vi "readEthernetLimitsFromXml.vi"(6 "type":string, 8 "error in (no error)":errorcluster, 9 "device.lvclass":refnum<class "device.lvclass">, 10 "xml in":refnum<class "NativeXML.lvclass">, 11 "deviceDataBase in":refnum<class "deviceDataBase.lvclass">) -> (0 "error out":errorcluster, 1 "device.lvclass out":refnum<class "device.lvclass">, 2 "xml out":refnum<class "NativeXML.lvclass">, 3 "deviceDataBase out":refnum<class "deviceDataBase.lvclass">)   [LabVIEW 2009, in "Tools.lvlib" / "DatabaseHelpers.lvlib" / "deviceDataBase.lvclass"]
uses:
  deviceDataBase.lvclass
  Database Objects/device/device.lvclass
  NativeXML/NativeXML.lvclass
  Database Objects/device/EthernetSupply/ethernetSupply.lvclass
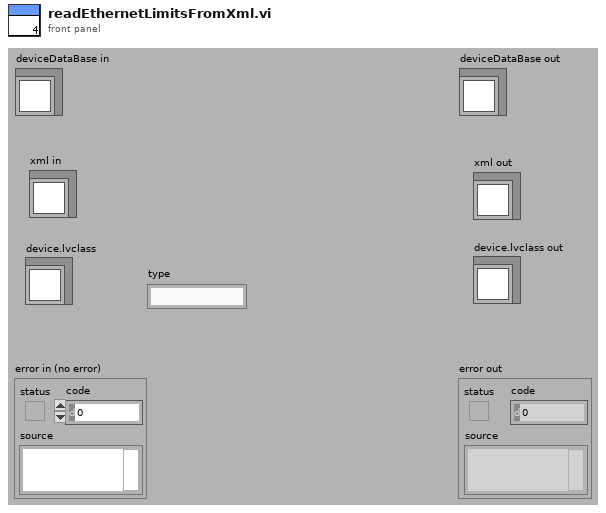
[diagram p1: front panel]
types:
  T1 = cluster{"Range":cluster{"units":string, "min":dbl, "max":dbl}, "triggering_inUse":cluster{"start_trigger":string, "clock":string}, "Limits":cluster{"VoltageLimit":dbl, "CurrentLimit":dbl}}[]
  T2 = cluster{"Range":cluster{"units":string, "min":dbl, "max":dbl}, "triggering_inUse":cluster{"start_trigger":string, "clock":string}, "Limits":cluster{"VoltageLimit":dbl, "CurrentLimit":dbl}}
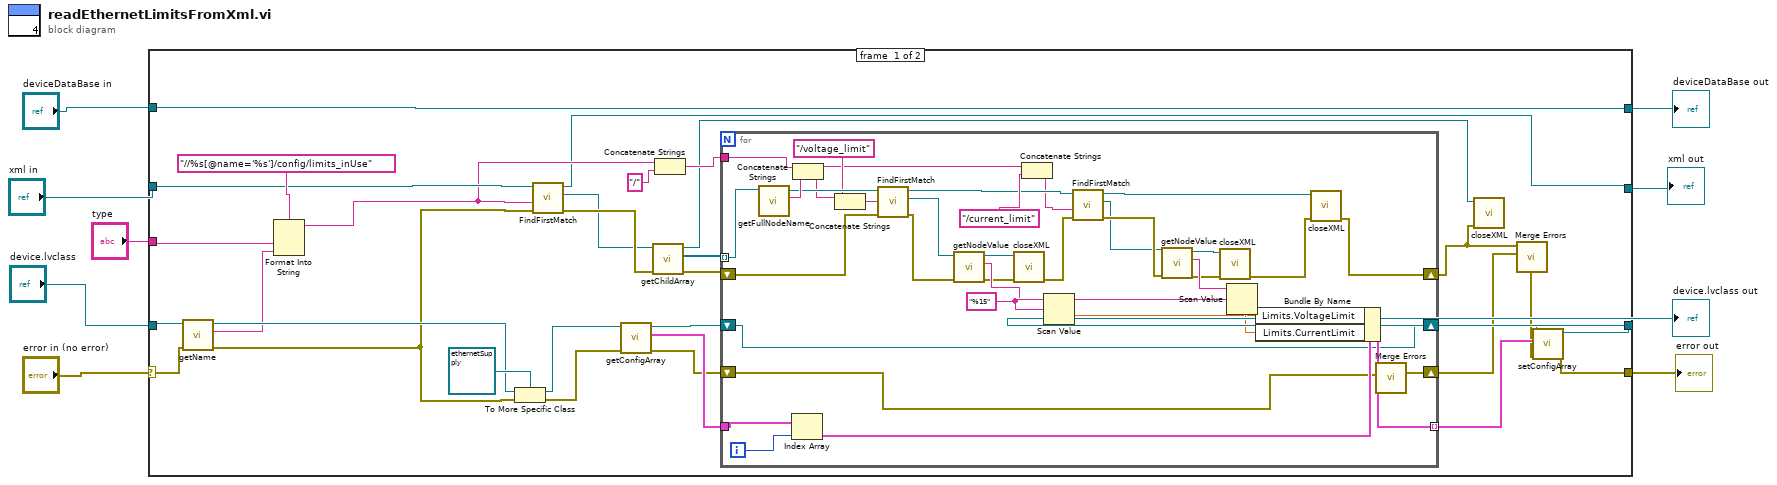
[diagram p0: block diagram]
diagram:
  n1 = case shown="No Error" "error in (no error)" {
    selector: "error in (no error)" -> [w23 w79]
    tunnel: [w30 w79] -> w7
    tunnel: [w40 w78] -> w8
    tunnel: "xml in" -> [w15 w77]
    tunnel: "device.lvclass" -> [w25 w76]
    tunnel: [w31 w76] -> w2
    tunnel: [w12 w77] -> w3
    tunnel: "deviceDataBase in" -> [w40 w78]
    tunnel: "type" -> [w22 _]
    frame #0 {
      n2 = call "getName.vi"("error in (no error)"=w23, "device.lvclass in"=w25) -> ("error out"=w14:errorcluster, "name"=w21:string, "device.lvclass out"=w24:refnum<class "device.lvclass">)  [unwired: 7 in]
      n3 = Format Into String(format string="//%s[@name='%s']/config/limits_inUse", w22, w21) -> (resulting string=w13:string)  [unwired: 2 in, 1 out]
      n4 = To More Specific Class(target class=refnum<class "ethernetSupply.lvclass"> refnum ("Tools.lvlib:DatabaseHelpers.lvlib:EthernetSupply.lvclass"), reference=w24, error in=w14) -> (specific class reference=w36:refnum<class "ethernetSupply.lvclass">, error out=w34:errorcluster)
      n5 = call "FindFirstMatch.vi"("error in (no error)"=w14, "xPath"=w13, "NativeXML in"=w15) -> ("error out"=w11:errorcluster, "NativeXML match"=w10:refnum<class "NativeXML.lvclass">, "NativeXML out"=w12:refnum<class "NativeXML.lvclass">)  [unwired: 6 in]
      n6 = call "getConfigArray.vi"("error in (no error)"=w34, "EthernetSupply in"=w36) -> ("error out"=w33:errorcluster, "ConfigArray"=w35:T1, "EthernetSupply out"=w37:refnum<class "ethernetSupply.lvclass">)  [unwired: 7 in]
      n7 = call "getChildArray.vi"("error in (no error)"=w11, "NativeXML in"=w10) -> ("error out"=w27:errorcluster, "childArray"=w29:refnum<class "NativeXML.lvclass">[], "NativeXML out"=w16:refnum<class "NativeXML.lvclass">)  [unwired: 7 in]
      n8 = Concatenate Strings(w13, "/") -> (w18:string)
      n9 = for {
        shift-right: [w70] -> w32
        shift-left: w37 -> [w70]
        shift-right: [w74] -> w26
        shift-left: w33 -> [w69]
        tunnel: w29 -> [w61] mode=indexing
        tunnel: w35 -> [w73]
        tunnel: [w75] -> w38 mode=indexing
        shift-right: [w55] -> w17
        shift-left: w27 -> [w53]
        tunnel: w18 -> [w62]
        i -> [w71]
        w68 = "%15"
        n10 = call "getFullNodeName.vi"("NativeXML in"=w61) -> ("fullName"=w63:string, "NativeXML out"=w54:refnum<class "NativeXML.lvclass">)  [unwired: 8 in, 1 out]
        n11 = Index Array(array=w73, index=w71) -> (element=w72:T2)
        n12 = Concatenate Strings(w62, w63) -> (w48:string)
        n13 = Concatenate Strings(w48, "/voltage_limit") -> (w49:string)
        n14 = call "FindFirstMatch.vi"("error in (no error)"=w53, "xPath"=w49, "NativeXML in"=w54) -> ("error out"=w52:errorcluster, "NativeXML match"=w51:refnum<class "NativeXML.lvclass">, "NativeXML out"=w45:refnum<class "NativeXML.lvclass">)  [unwired: 6 in]
        n15 = call "getNodeValue.vi"("error in (no error)"=w52, "NativeXML in"=w51) -> ("error out"=w59:errorcluster, "Value"=w65:string, "NativeXML out"=w60:refnum<class "NativeXML.lvclass">)  [unwired: 7 in]
        n16 = call "closeXML.vi"("error in (no error)"=w59, "NativeXML in"=w60) -> ("error out"=w43:errorcluster)  [unwired: 9 in]
        n17 = Concatenate Strings(w48, "/current_limit") -> (w44:string)
        n18 = Scan Value(string=w65, format string=w68) -> (value=w66:dbl)  [unwired: 1 in, 1 out]
        n19 = call "FindFirstMatch.vi"("error in (no error)"=w43, "xPath"=w44, "NativeXML in"=w45) -> ("error out"=w42:errorcluster, "NativeXML match"=w41:refnum<class "NativeXML.lvclass">, "NativeXML out"=w46:refnum<class "NativeXML.lvclass">)  [unwired: 6 in]
        n20 = call "getNodeValue.vi"("error in (no error)"=w42, "NativeXML in"=w41) -> ("error out"=w58:errorcluster, "Value"=w64:string, "NativeXML out"=w57:refnum<class "NativeXML.lvclass">)  [unwired: 7 in]
        n21 = call "closeXML.vi"("error in (no error)"=w58, "NativeXML in"=w57) -> ("error out"=w56:errorcluster)  [unwired: 9 in]
        n22 = Scan Value(string=w64, format string=w68) -> (value=w67:dbl)  [unwired: 1 in, 1 out]
        n23 = Bundle By Name(cluster=w72, "Limits.VoltageLimit"=w66, "Limits.CurrentLimit"=w67) -> (w75:T2)
        n24 = call "closeXML.vi"("error in (no error)"=w56, "NativeXML in"=w46) -> ("error out"=w55:errorcluster)  [unwired: 9 in]
        n25 = call <vilib>:"Merge Errors.vi"("error in 2 (no error)"=w69) -> ("error out"=w74:errorcluster)  [unwired: 6 in]
      }
      n26 = call "closeXML.vi"("error in (no error)"=w17, "NativeXML in"=w16) -> ()  [unwired: 9 in, 1 out]
      n27 = call <vilib>:"Merge Errors.vi"("error in 2 (no error)"=w26, "error in 1 (no error)"=w17) -> ("error out"=w28:errorcluster)  [unwired: 5 in]
      n28 = call "setConfigArray.vi"("error in (no error)"=w28, "ConfigArray"=w38, "EthernetSupply in"=w32) -> ("error out"=w30:errorcluster, "EthernetSupply out"=w31:refnum<class "ethernetSupply.lvclass">)  [unwired: 7 in]
    }
    frame #1 {
    }
  }
  "error out" <- w7
  "deviceDataBase out" <- w8
  "xml out" <- w3
  "device.lvclass out" <- w2
